vi "Subscribe.vi"(0 "error in":errorcluster, 2 "Topic":string="/junk", 3 "node":string) -> (1 "error out":errorcluster, 4 "Reply":string)   [LabVIEW 2015]
uses:
  ROS/Code/SubVIs/_ROSDirection.ctl
  ROS/MessageParsing/std_msgs/subs/parse_string_scalar.vi
panel:
  # "Register subscriber"
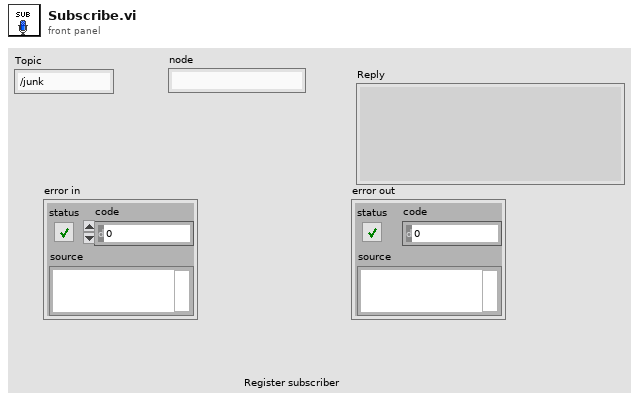
[diagram p1: front panel]
types:
  T1 = typedef "_ROSDirection.ctl" = enum16{"Node", "Publisher", "Subscriber", "ServiceClient", "ServiceProvider"}
  T2 = cluster{"Topic":string, "Type":string, "Action":T1, "Update (ms)":u16, "queue":u16}
  T3 = typedef "_ROSControl.ctl" = cluster{"topic port":u16, "Node":string, "topic":string, "type":string, "node port":u16, "error ":errorcluster, "Direction":T1, "Update (ms)":u16, "FIFO size":u16}
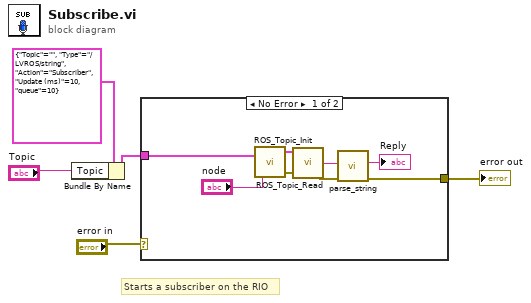
[diagram p0: block diagram]
diagram:
  # "Starts a subscriber on the RIO"
  n1 = Bundle By Name(cluster=T2 {"Topic"="", "Type"="/LVROS/string", "Action"=enum."Subscriber", "Update (ms)"=10, "queue"=10} ("Definitions"), "Topic"="Topic") -> (w4:T2)
  n2 = case shown="No Error" "error in" {
    selector: "error in" -> [_ w14]
    tunnel: w4 -> [w10 _]
    tunnel: [w8 w14] -> w2
    frame No Error {
      n3 = call "ROS_Topic_Init.vi"("Definitions"=w10, "node"="node") -> ("ROS out"=w13:T3, "error out"=w7:errorcluster)  [unwired: 1 in]
      n4 = call "ROS_Topic_Read.vi"("error in (no error)"=w7, "ROS in"=w13) -> ("error out"=w6:errorcluster, "Reply"=w11:string)  [unwired: 1 in, 1 out]
      n5 = call-poly "parse_string.vi"("error in"=w6, "msg in"=w11) -> ("error out"=w8:errorcluster, "string"=→"Reply":string)  [unwired: 3 in, 1 out]
    }
    frame Error {
    }
  }
  "error out" <- w2
